vi "XML_Get_Data.vi"(10 "XML Data to Retrieve":T1(ring), 11 "XML String":string) -> (1 "XML String Array":string[](array[string]), 2 "XML Data":string[](array[string]), 3 "XML Lines":string[](array[string]))   [LabVIEW 2011]
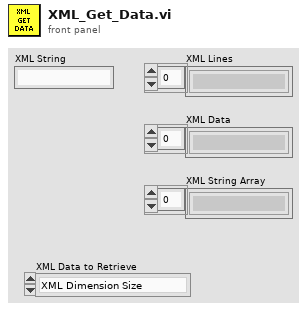
[diagram p1: front panel]
types:
  T1 = enum16{"XML Dimension Size", "XML Name", "XML Value"}
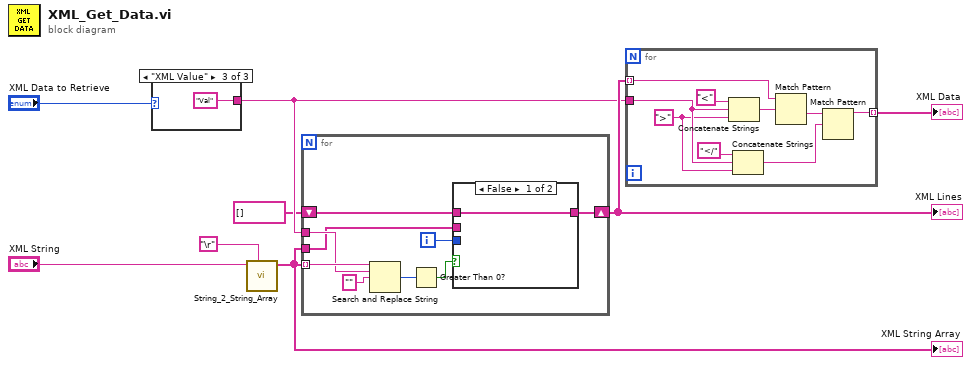
[diagram p0: block diagram]
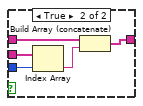
[diagram p2: hidden frame]
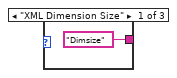
[diagram p3: hidden frame]
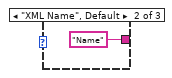
[diagram p4: hidden frame]
diagram:
  n1 = case shown="\"XML Value\"" "XML Data to Retrieve" {
    tunnel: ["Dimsize" ("search string") "Name" ("search string") "Val" ("search string")] -> w4
    frame "XML Dimension Size" {
    }
    frame "XML Name", Default {
    }
    frame "XML Value" {
    }
  }
  n2 = call "String_2_String_Array.vi"("delimiter (;)"="\r", "String"="XML String") -> ("String Array"=w6:string[])  [unwired: 9 in]
  "XML String Array" <- w6
  n3 = for {
    tunnel: w6 -> [w20] mode=indexing
    tunnel: w4 -> [w17]
    tunnel: w6 -> [w14]
    shift-right: [w13] -> w7
    shift-left: string[] [] -> [w12]
    i -> [w15]
    n4 = Search and Replace String(input string=w20, search string=w17, replace string="" ("replace string (\"\")")) -> (number of replacements=w18:i32)  [unwired: 5 in, 3 out]
    n5 = Greater Than 0?(x=w18) -> (x > 0?=w16:bool)
    n6 = case shown="False" w16 {
      tunnel: w15 -> [_ w26]
      tunnel: w14 -> [_ w25]
      tunnel: [w21 w23] -> w13
      tunnel: w12 -> [w21 w22]
      frame False {
      }
      frame True {
        n7 = Index Array(array=w25, index=w26) -> (element=w24:string)
        n8 = Build Array (concatenate)(w22, w24) -> (w23:string[])
      }
    }
  }
  "XML Lines" <- w7
  n9 = for {
    tunnel: w4 -> [w35]
    tunnel: w7 -> [w34] mode=indexing
    tunnel: [w27] -> w8 mode=indexing
    w30 = ">" ("string")
    n10 = Concatenate Strings("<" ("string"), w35, w30) -> (w33:string)
    n11 = Concatenate Strings("</" ("string"), w35, w30) -> (w28:string)
    n12 = Match Pattern(string=w34, regular expression=w33) -> (after substring=w32:string)  [unwired: 1 in, 3 out]
    n13 = Match Pattern(string=w32, regular expression=w28) -> (before substring=w27:string)  [unwired: 1 in, 3 out]
  }
  "XML Data" <- w8
